vi "Lookup Channel.vi"(8 "error in (no error)":errorcluster, 10 "Channel Name":string, 11 "Group in":refnum<class "Group.lvclass">) -> (0 "error out":errorcluster, 2 "Channel":refnum<class "Channel.lvclass">, 3 "Group out":refnum<class "Group.lvclass">)   [LabVIEW 2020, in "Vecto.lvlib" / "Group.lvclass"]
uses:
  Group.lvclass
  Channel/Channel.lvclass
  Group.lvclass/Group.ctl
  Group Config/Group Config.lvclass
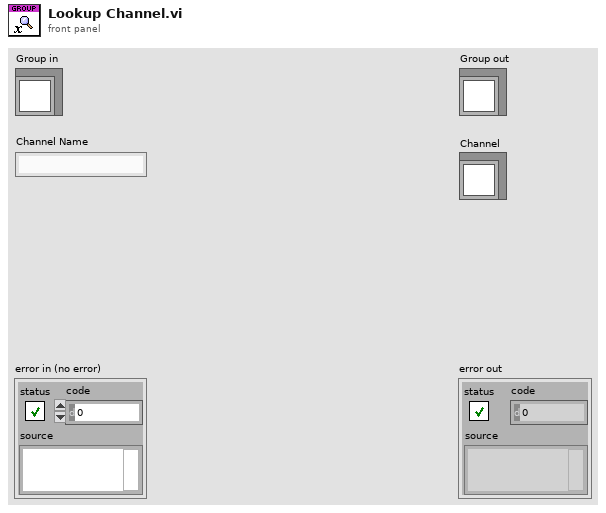
[diagram p1: front panel]
types:
  T1 = typedef "Vecto.lvlib/Group.lvclass/Ref.ctl" = cluster{"Channel Index Map":map{string, i32}, "Channel Info":T2[], "Scaled":dbl[], "Timestamp":dbl[], "Raw":dbl[]}
  T2 = typedef "Vecto.lvlib/Channel Info.ctl" = cluster{"Name":string, "Group":string, "Owning Node":string, "Owning Task":string, "Resource":string}
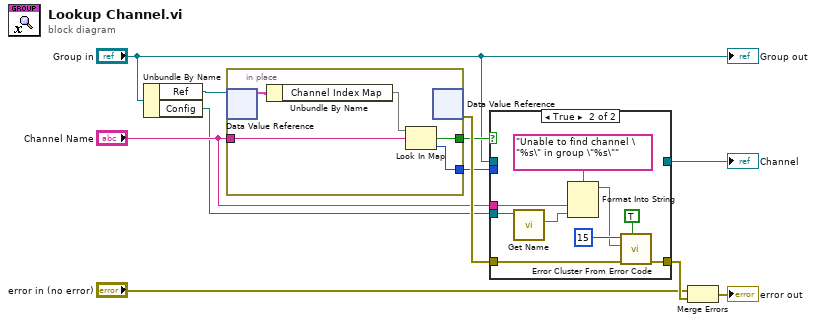
[diagram p0: block diagram]
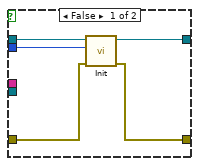
[diagram p2: hidden frame]
diagram:
  n1 = Unbundle By Name("Group in") -> ("Ref"=w10:refnum<data-value>, "Config"=w7:refnum<class "Group Config.lvclass">)
  n2 = in-place {
    in-place-border: "Channel Name" -> [w14]
    in-place-border: [w13] -> w9
    in-place-border: [w12] -> w2
    n3 = in-place-dvr #1(w10) -> (w16:T1)  [unwired: 1 out]
    n4 = Unbundle By Name(w16) -> ("Channel Index Map"=w15:map{string, i32})
    n5 = Look In Map(map=w15, key=w14) -> (key not found?=w13:bool, value=w12:i32)  [unwired: 1 in]
    n6 = in-place-dvr #1() -> (w11:errorcluster)  [unwired: 1 in, 1 out]
  }
  n7 = case shown="True" w9 {
    tunnel: w11 -> [w21 w30]
    tunnel: "Channel Name" -> [_ w27]
    tunnel: w7 -> [_ w24]
    tunnel: [w20 w23] -> w6
    tunnel: [w19 _] -> w3
    tunnel: w2 -> [w18 _]
    tunnel: "Group in" -> [w17 _]
    frame False {
      n8 = call "Init.vi"("error in (no error)"=w21, "Channel Index"=w18, "Group"=w17) -> ("error out"=w20:errorcluster, "Channel out"=w19:refnum<class "Channel.lvclass">)  [unwired: 7 in]
    }
    frame True {
      n9 = call "Get Name.vi"("Group Config in"=w24) -> ("Name"=w22:string)  [unwired: 8 in, 2 out]
      n10 = Format Into String(format string="Unable to find channel \"%s\" in group \"%s\"", w27, w22) -> (resulting string=w26:string)  [unwired: 2 in, 1 out]
      n11 = call <vilib>:"Error Cluster From Error Code.vi"("show call chain? (False)"=TRUE, "error in (no error)"=w30, "error message (\"\")"=w26, "error code (0)"=15) -> ("error out"=w23:errorcluster)  [unwired: 5 in]
    }
  }
  "Channel" <- w3
  n12 = Merge Errors("error in (no error)", w6) -> (→"error out":errorcluster)
  "Group out" <- "Group in"
